vi "Get QueryRequest.vi"(8 "error in (no error)":errorcluster, 11 "gRPCid":T2) -> (0 "error out":errorcluster, 2 "Request Data":T1, 3 "gRPCid out":T2)   [LabVIEW 2019]
uses:
  gRPC interface/Server API/typeDefs/grpcId.ctl
  QueryRequest_Data.ctl
  0f811efc-ff8c-4c07-a6dc-77b3b05bf966.vi
  gRPC interface/gprc-lvsupport.lvlib
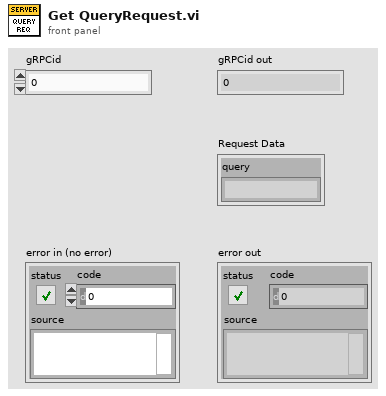
[diagram p1: front panel]
types:
  T1 = typedef "QueryRequest_Data.ctl" = cluster{"query":string}
  T2 = typedef "gprc-lvsupport.lvlib/grpcId.ctl" = u64
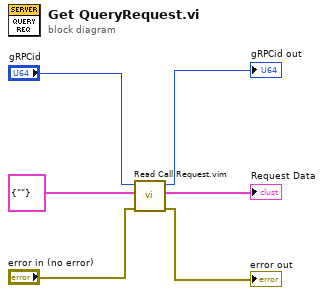
[diagram p0: block diagram]
diagram:
  n1 = call "Read Call Request.vim"("error in (no error)"="error in (no error)", "Data Type"=T1 {"query"=""} ("QueryRequst_Data"), "gRPCid in"="gRPCid") -> ("error out"=→"error out":errorcluster, "Request Data"=→"Request Data":T1, "gRPCid out"=→"gRPCid out":T2)  [unwired: 6 in]
